vi "FiltroSubVi(examen1).vi"(11 "Numeric in":dbl) -> (3 "Numeric":dbl)   [LabVIEW 2020]
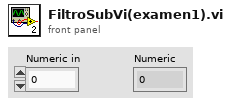
[diagram p1: front panel]
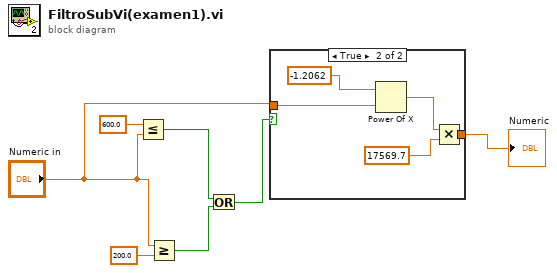
[diagram p0: block diagram]
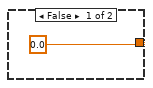
[diagram p2: hidden frame]
diagram:
  n1 = Less Or Equal?(x=600.0, y="Numeric in") -> (x <= y?=w5:bool)
  n2 = Greater Or Equal?(x="Numeric in", y=200.0) -> (x >= y?=w4:bool)
  n3 = Or(x=w5, y=w4) -> (x .or. y?=w3:bool)
  n4 = case shown="True" w3 {
    tunnel: "Numeric in" -> [_ w10]
    tunnel: [0.0 w9] -> w1
    frame False {
    }
    frame True {
      n5 = Power Of X(1:w10, 2:-1.2062 ("x")) -> (0:w12:dbl)
      n6 = Multiply(x=w12, y=17569.7) -> (x*y=w9:dbl)
    }
  }
  "Numeric" <- w1
